vi "RT led test.vi"() -> ()   [LabVIEW 2015]
uses:
  <vilib>/FPGAPlugInAG/cRIO-9118/niLvFpga_Open_cRIO-9118.vi
  <vilib>/rvi/interface/common/dynamic/niFpgaDynamicAddResources.vi
  <vilib>/Utility/error.llb/Error Cluster From Error Code.vi
  <vilib>/rvi/errors/niLvFpgaAdjustHostInterfaceError.vi
  <vilib>/FPGAPlugInAG/Dynamic/niLvFpga_Close_Dynamic.vi
  <vilib>/rvi/interface/nirviOpenFPGA/nirviOpenFPGA.xnode
  FPGA Bitfiles/LEDcontrol_FPGATarget_FPGAuploaddatato_WiOhyWI+G-E.lvbitx
  FPGA upload data to LEDs.vi
  <vilib>/rvi/interface/nirviMethod/nirviMethod.xnode
  <vilib>/rvi/interface/nirviCloseFPGA/nirviCloseFPGA.xnode
  <vilib>/rvi/errors/niLvFpgaMergeErrorWithErrorCode.vi
  <vilib>/FPGAPlugInAG/Dynamic/niLvFpga_WriteFifo_Dynamic.vi
panel:
  in  "Pattern":string(combo)="One white"
  in  "Wire ID":u32=1 format="%.0x"
  out "Iteration ms":u32=20
  in  "ms delay":u32=50
  out "LEDs":u32[](array[colorbox])=[56797, 1172948, 2223306, 3338688, 4388532, 5438120, 6487451, 7470734, 8388479, 9371249, 10222946, 11074130, 11859522, 12644658, 13298721, 13952273, 14540032, 15062033, 15518241, 15843378, 16168002, 16427090, 16620386, 16682609, 16744320, 16675214, 16605851, 16405160, 16138932, 15807168, 15475146, 15012308, 14483677, 13898213, 13246956, 12595953, 11813622, 11031290, 10183421, 9335294, 8356095, 7442174, 6462461, 5417210, 4371702, 3326193, 2214636, 1168613]
  in  "stop":bool
  # "WS2812 control example"
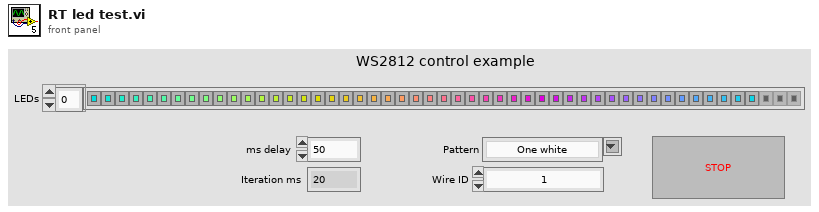
[diagram p1: front panel]
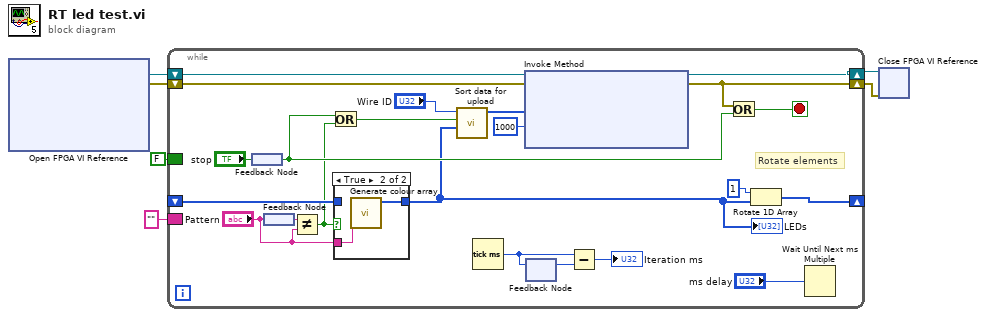
[diagram p0: block diagram]
diagram:
  n1 = xnode "Open FPGA VI Reference"() -> ("FPGA VI Reference Out"=w6:refnum<k20>, "error out"=w5:errorcluster)  [unwired: 2 in]
  n2 = while {
    shift-right: [w20] -> w3
    shift-left: w5 -> [w27]
    shift-right: [w28] -> w4
    shift-left: w6 -> [w26]
    shift-right: [w25] -> _
    shift-left: _ -> [w11]
    border: FALSE ("stop") -> [_]
    border: "" ("Pattern") -> [_]
    stop <- w21 stop-if-true
    # "Rotate elements"
    n3 = feedback-in #1("stop") -> ()
    n4 = feedback #1() -> (w15:bool)
    n5 = feedback-in #2("Pattern") -> ()
    n6 = feedback #2() -> (w12:string)
    n7 = Not Equal?(x=w12, y="Pattern") -> (x != y?=w7:bool)
    n8 = Or(x=w15, y=w7) -> (x .or. y?=w8:bool)
    n9 = case shown="True" w7 {
      tunnel: [w29 w31] -> w10
      tunnel: w11 -> [w29 _]
      tunnel: "Pattern" -> [_ w30]
      frame False {
      }
      frame True {
        n10 = call "Generate colour array.vi"("Combo Box"=w30) -> ("Array"=w31:u32[])  [unwired: 10 in]
      }
    }
    "LEDs" <- w10
    n11 = call "Sort data for upload.vi"("Colour array in"=w10, "Zero Outputs?"=w8, "ID"="Wire ID") -> ("Upload data"=w14:u32[])  [unwired: 8 in]
    n12 = Tick Count (ms)() -> (millisecond timer value=w18:u32)
    n13 = xnode "Invoke Method"("FPGA VI Reference In"=w26, "error in"=w27, "Data"=w14, "Timeout (ms)"=1000) -> ("FPGA VI Reference Out"=w28:refnum<k20>, "error out"=w20:errorcluster)  [unwired: 1 out]
    n14 = feedback-in #3(w18) -> ()
    n15 = feedback #3() -> (w19:u32)  [unwired: 1 in]
    n16 = Subtract(x=w18, y=w19) -> (x-y=→"Iteration ms":u32)
    n17 = Or(x=w20, y=w15) -> (x .or. y?=w21:bool)
    n18 = Rotate 1D Array(1:w10, 2:1 ("n")) -> (0:w25:u32[])
    n19 = Wait Until Next ms Multiple(millisecond multiple="ms delay") -> ()  [unwired: 1 out]
  }
  n20 = xnode "Close FPGA VI Reference"("FPGA VI Reference In"=w4, "error in"=w3) -> ()  [unwired: 1 out]
